vi "April 2019 SubGR.vi"(0 "Folder Name":string, 1 "Name of File":string, 2 "Folder to Save":path, 3 "Timepoints":dbl[](array[numeric]), 4 "Vx array":dbl[](array[numeric]), 5 "Vy array":dbl[](array[numeric])) -> ()   [LabVIEW 2014]
uses:
  <vilib>/Utility/file.llb/Write Delimited Spreadsheet (DBL).vi
  <vilib>/Utility/file.llb/Read Delimited Spreadsheet (DBL).vi
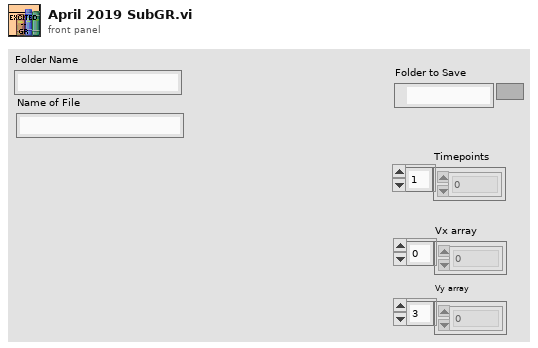
[diagram p1: front panel]
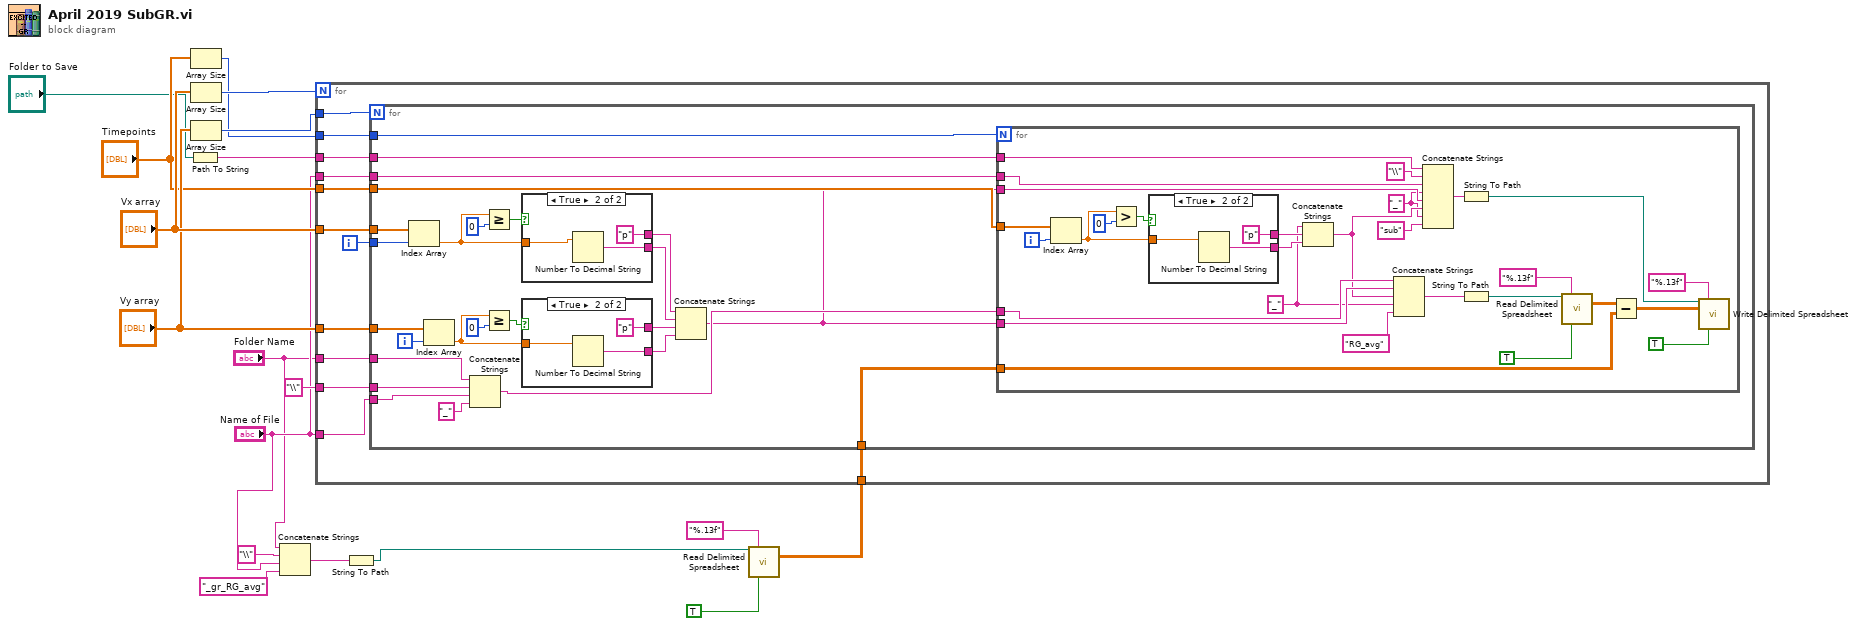
[diagram p0: block diagram]
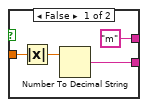
[diagram p2: hidden frame]
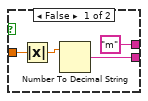
[diagram p3: hidden frame]
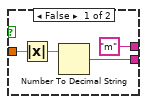
[diagram p4: hidden frame]
diagram:
  n1 = Path To String(path="Folder to Save") -> (string=w11:string)
  n2 = Array Size(array="Timepoints") -> (size(s)=w15:i32)
  n3 = Array Size(array="Vx array") -> (size(s)=w17:i32)
  n4 = Array Size(array="Vy array") -> (size(s)=w16:i32)
  n5 = Concatenate Strings("Folder Name", "\\" ("string"), "Name of File", "_gr_RG_avg" ("string")) -> (w3:string)
  n6 = String To Path(string=w3) -> (path=w2:path)
  n7 = call-poly <vilib>:"Read Delimited Spreadsheet.vi"("file path (dialog if empty)"=w2, "format (%.3f)"="%.13f", "transpose? (F)"=TRUE) -> ("all rows"=w8:dbl[][])  [unwired: 7 in, 5 out]
  n8 = for {
    N: w17 -> [_]
    tunnel: "Name of File" -> [w30]
    tunnel: "\\" -> [w29]
    tunnel: "Folder Name" -> [w28]
    tunnel: w16 -> [w27]
    tunnel: w15 -> [w26]
    tunnel: "Vx array" -> [w25]
    tunnel: "Vy array" -> [w23]
    tunnel: "Timepoints" -> [w22]
    tunnel: w11 -> [w21]
    tunnel: "Name of File" -> [w20]
    tunnel: w8 -> [w19]
    i -> [w24]
    n9 = for {
      N: w27 -> [_]
      tunnel: w30 -> [w32]
      tunnel: w29 -> [w33]
      tunnel: w28 -> [w55]
      tunnel: w26 -> [w54]
      tunnel: w25 -> [w50]
      tunnel: w24 -> [w51]
      tunnel: w23 -> [w45]
      tunnel: w22 -> [w39]
      tunnel: w21 -> [w38]
      tunnel: w20 -> [w37]
      tunnel: w19 -> [w31]
      i -> [w44]
      n10 = Index Array(array=w50, index=w51) -> (element=w49:dbl)
      n11 = Index Array(array=w45, index=w44) -> (element=w46:dbl)
      n12 = Concatenate Strings(w55, w33, w32, "_") -> (w35:string)
      n13 = Greater Or Equal?(x=w49, y=0) -> (x >= y?=w52:bool)
      n14 = Greater Or Equal?(x=w46, y=0) -> (x >= y?=w48:bool)
      n15 = case shown="True" w52 {
        tunnel: ["m" "p"] -> w43
        tunnel: w49 -> [w65 w67]
        tunnel: [w63 w68] -> w42
        frame False {
          n16 = Absolute Value(x=w65) -> (abs(x)=w64:dbl)
          n17 = Number To Decimal String(number=w64) -> (decimal integer string=w63:string)  [unwired: 1 in]
        }
        frame True {
          n18 = Number To Decimal String(number=w67) -> (decimal integer string=w68:string)  [unwired: 1 in]
        }
      }
      n19 = case shown="True" w48 {
        tunnel: ["m" "p"] -> w41
        tunnel: w46 -> [w58 w60]
        tunnel: [w56 w61] -> w40
        frame False {
          n20 = Absolute Value(x=w58) -> (abs(x)=w57:dbl)
          n21 = Number To Decimal String(number=w57) -> (decimal integer string=w56:string)  [unwired: 1 in]
        }
        frame True {
          n22 = Number To Decimal String(number=w60) -> (decimal integer string=w61:string)  [unwired: 1 in]
        }
      }
      n23 = Concatenate Strings(w43, w42, w41, w40) -> (w34:string)
      n24 = for {
        N: w54 -> [_]
        tunnel: w39 -> [w95]
        tunnel: w38 -> [w90]
        tunnel: w37 -> [w87]
        tunnel: w35 -> [w81]
        tunnel: w34 -> [w80]
        tunnel: w31 -> [w76]
        tunnel: w34 -> [w74]
        i -> [w94]
        w79 = "_"
        w72 = "_" ("string")
        n25 = Index Array(array=w95, index=w94) -> (element=w97:dbl)
        n26 = Greater?(x=w97, y=0) -> (0:w96:bool)
        n27 = case shown="True" w96 {
          tunnel: ["m" "p"] -> w92
          tunnel: w97 -> [w101 w103]
          tunnel: [w99 w104] -> w93
          frame False {
            n28 = Absolute Value(x=w101) -> (abs(x)=w100:dbl)
            n29 = Number To Decimal String(number=w100) -> (decimal integer string=w99:string)  [unwired: 1 in]
          }
          frame True {
            n30 = Number To Decimal String(number=w103) -> (decimal integer string=w104:string)  [unwired: 1 in]
          }
        }
        n31 = Concatenate Strings(w79, w92, w93) -> (w73:string)
        n32 = Concatenate Strings(w81, w80, w73, w79, "RG_avg") -> (w83:string)
        n33 = Concatenate Strings(w90, "\\" ("string"), w87, w72, w74, w73, w72, "sub" ("string")) -> (w70:string)
        n34 = String To Path(string=w70) -> (path=w89:path)
        n35 = String To Path(string=w83) -> (path=w84:path)
        n36 = call-poly <vilib>:"Read Delimited Spreadsheet.vi"("file path (dialog if empty)"=w84, "format (%.3f)"="%.13f", "transpose? (F)"=TRUE) -> ("all rows"=w77:dbl[][])  [unwired: 7 in, 5 out]
        n37 = Subtract(x=w77, y=w76) -> (x-y=w75:dbl[][])
        n38 = call-poly <vilib>:"Write Delimited Spreadsheet.vi"("file path (dialog if empty)"=w89, "format (%.3f)"="%.13f", "2D data"=w75, "transpose? (F)"=TRUE) -> ()  [unwired: 10 in, 2 out]
      }
    }
  }
